vi "Build Window Title.vi"(9 "Root Window Title":string, 10 "Saved Notebook?":bool, 11 "File Path in":path) -> (1 "Modified Window Title":string)   [LabVIEW 2019, in "Notebook.lvlib"]
uses:
  Notebook.lvlib
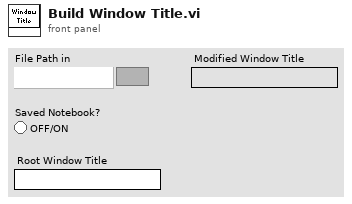
[diagram p1: front panel]
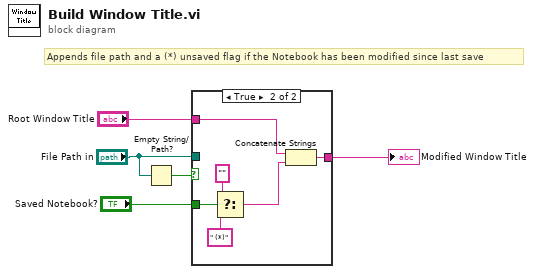
[diagram p0: block diagram]
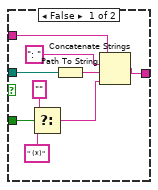
[diagram p2: hidden frame]
diagram:
  # "Appends file path and a (*) unsaved flag if the Notebook has been modified since last save"
  n1 = Empty String/Path?(string/path="File Path in") -> (empty?=w1:bool)
  n2 = case shown="True" w1 {
    tunnel: [w14 w20] -> w5
    tunnel: "Root Window Title" -> [w11 w17]
    tunnel: "Saved Notebook?" -> [w9 w15]
    tunnel: "File Path in" -> [w6 _]
    frame False {
      n3 = Select(t="" ("string"), s=w9, f=" (*)" ("string")) -> (s? t:f=w10:string)
      n4 = Path To String(path=w6) -> (string=w8:string)
      n5 = Concatenate Strings(w11, ": " ("string"), w8, w10) -> (w14:string)
    }
    frame True {
      n6 = Select(t="" ("string"), s=w15, f=" (*)" ("string")) -> (s? t:f=w16:string)
      n7 = Concatenate Strings(w17, w16) -> (w20:string)
    }
  }
  "Modified Window Title" <- w5
